vi "Plot default grid colors.vi"(5 "Major Color visible?":bool, 7 "Minor Color visible?":bool, 9 "Minor Color":u32, 11 "Major Color":u32) -> (1 "Minor Color":u32, 3 "Major Color":u32)   [LabVIEW 2021, in "RocketPlot.lvlib"]
uses:
  RocketPlot.lvlib
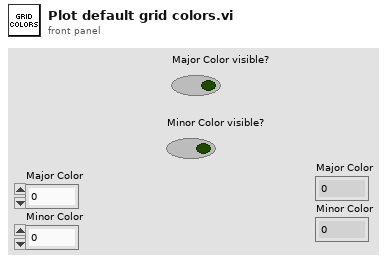
[diagram p1: front panel]
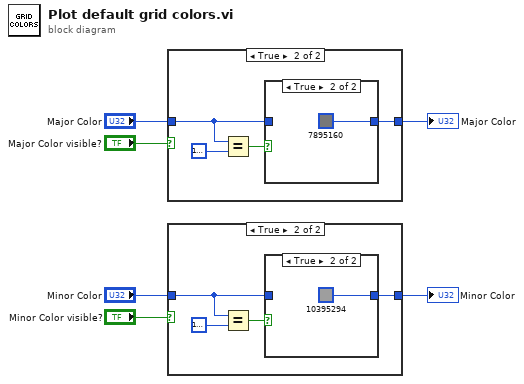
[diagram p0: block diagram]
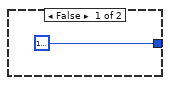
[diagram p2: hidden frame]
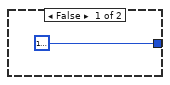
[diagram p4: hidden frame]
diagram:
  n1 = case shown="True" "Major Color visible?" {
    tunnel: "Major Color" -> [_ w8]
    tunnel: [u32 16777216 w9] -> w2
    frame False {
    }
    frame True {
      n2 = Equal?(x=w8, y=u32 16777216) -> (x = y?=w10:bool)
      n3 = case shown="True" w10 {
        tunnel: [w12 u32 7895160] -> w9
        tunnel: w8 -> [w12 _]
        frame False {
        }
        frame True {
        }
      }
    }
  }
  "Major Color" <- w2
  n4 = case shown="True" "Minor Color visible?" {
    tunnel: "Minor Color" -> [_ w15]
    tunnel: [u32 16777216 w16] -> w1
    frame False {
    }
    frame True {
      n5 = Equal?(x=w15, y=u32 16777216) -> (x = y?=w17:bool)
      n6 = case shown="True" w17 {
        tunnel: [w19 u32 10395294] -> w16
        tunnel: w15 -> [w19 _]
        frame False {
        }
        frame True {
        }
      }
    }
  }
  "Minor Color" <- w1
